vi "stop.vi"(8 "error in (no error)":errorcluster, 11 "Model in":refnum<class "Model.lvclass">) -> (0 "error out":errorcluster, 3 "Model out":refnum<class "Model.lvclass">)   [LabVIEW 2015, in "Model.lvclass"]
uses:
  Model.lvclass
  Model.lvclass/Model.ctl
  <userlib>/Common/ILC/ILC/ILC.lvclass
  <userlib>/Common/Devices/DistanceGauge/DistanceGauge/DistanceGauge.lvclass
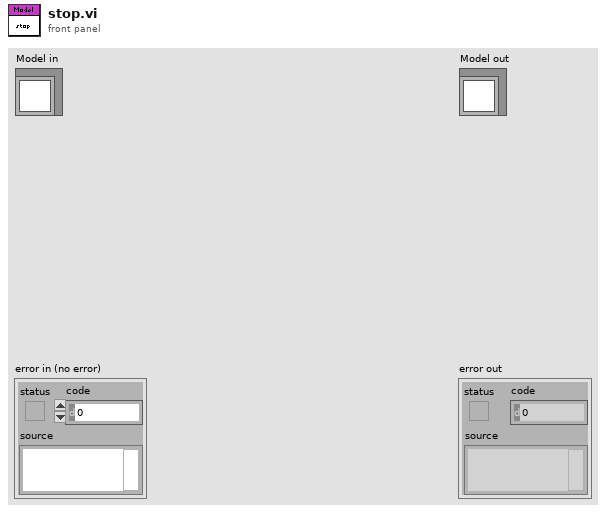
[diagram p1: front panel]
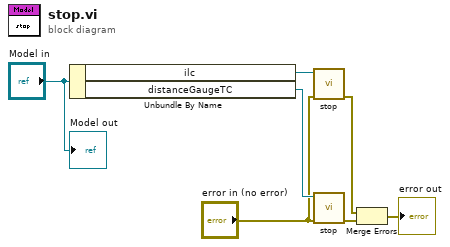
[diagram p0: block diagram]
diagram:
  n1 = Unbundle By Name("Model in") -> ("ilc"=w6:refnum<class "ILC.lvclass">, "distanceGaugeTC"=w5:refnum<class "DistanceGaugeTC.lvclass">)
  n2 = call <userlib>:"stop.vi"("error in (no error)"="error in (no error)", "ILC in"=w6) -> ("error out"=w3:errorcluster)  [unwired: 8 in, 1 out]
  n3 = call <userlib>:"stop.vi"("error in (no error)"="error in (no error)", "DistanceGauge in"=w5) -> ("error out"=w2:errorcluster)  [unwired: 8 in, 1 out]
  n4 = Merge Errors(w3, w2) -> (→"error out":errorcluster)
  "Model out" <- "Model in"
